vi "signal_1(SubVI).vi"(11 "x":dbl) -> (3 "Numeric":dbl)   [LabVIEW 2014]
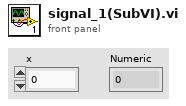
[diagram p1: front panel]
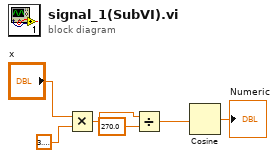
[diagram p0: block diagram]
diagram:
  n1 = Multiply(x="x", y=3.141592653589793) -> (x*y=w5:dbl)
  n2 = Divide(x=w5, y=270.0) -> (x/y=w3:dbl)
  n3 = Cosine(x=w3) -> (cos(x)=→"Numeric":dbl)
